vi "保存文件头.vi"(0 "error in (no error)":errorcluster caption="错误输入（无错误）", 1 "转角起点":dbl, 2 "转角终点":dbl, 3 "转角速度":dbl, 5 "实际备注数组":string[](array[string]), 7 "数据存储路径":path, 9 "采样率":u32, 11 "测试类型":dbl, 12 "单位":string, 13 "气压":dbl) -> (4 "error out":errorcluster caption="错误输出", 6 "引用句柄输出":refnum<file>, 15 "实际存储路径":path caption="新建文件路径（取消时为非法路径）")   [LabVIEW 2016]
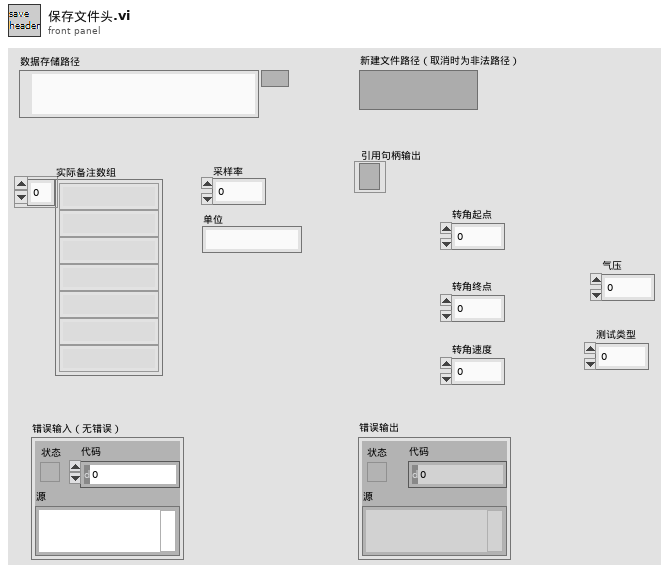
[diagram p1: front panel]
types:
  T1 = enum16{"open", "replace", "create", "open or create", "replace or create", "replace or create with confirmation"}
  T2 = cluster{"seconds since 1Jan1904":timestamp, "采样率":u32, "单位":string, "实际备注数组":string[], "转角终点":dbl, "转角起点":dbl, "转角速度":dbl, "测试类型":dbl, "气压":dbl}
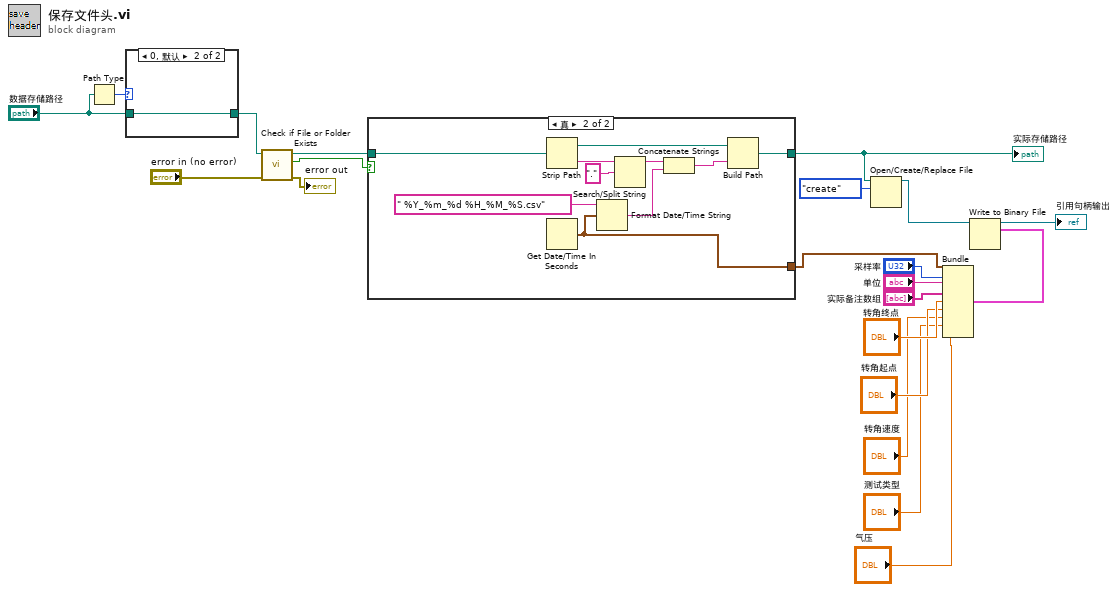
[diagram p0: block diagram]
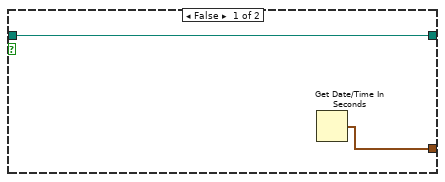
[diagram p2: hidden frame]
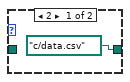
[diagram p3: hidden frame]
diagram:
  n1 = Path Type(1:"数据存储路径") -> (0:w21:i16)
  n2 = case shown="0, 默认" w21 {
    tunnel: "数据存储路径" -> [_ w23]
    tunnel: [path "c:/data.csv" w23] -> w17
    frame 2 {
    }
    frame 0, Default {
    }
  }
  n3 = call <vilib>:"Check if File or Folder Exists.vi"("error in (no error)"="error in (no error)", "path"=w17) -> ("error out"=→"error out":errorcluster, "file or folder exists?"=w18:bool, "dup path"=w19:path)  [unwired: 7 in]
  n4 = case shown="真" w18 {
    tunnel: w19 -> [w25 w35]
    tunnel: [w25 w27] -> w14
    tunnel: [w24 w26] -> w8
    frame False {
      n5 = Get Date/Time In Seconds() -> (seconds since 1Jan1904=w24:timestamp)
    }
    frame True {
      n6 = Strip Path(path=w35) -> (stripped path=w29:path, name=w32:string)
      n7 = Get Date/Time In Seconds() -> (seconds since 1Jan1904=w26:timestamp)
      n8 = Format Date/Time String(time format string (%c)=" %Y_%m_%d %H_%M_%S.csv" ("时间格式字符串(%c)"), seconds (now)=w26) -> (date/time string=w33:string)  [unwired: 1 in]
      n9 = Search/Split String(string=w32, search string/char (-)="." ("搜索字符串/字符(-)")) -> (substring before match=w30:string)  [unwired: 1 in, 2 out]
      n10 = Concatenate Strings(w30, w33) -> (w28:string)
      n11 = Build Path(base path=w29, name or relative path=w28) -> (appended path=w27:path)
    }
  }
  "实际存储路径" <- w14
  n12 = Open/Create/Replace File(file path (use dialog)=w14, operation (0:open)=T1."create" ("操作(0:open)")) -> (refnum out=w7:refnum<file>)  [unwired: 4 in, 2 out]
  n13 = Bundle("seconds since 1Jan1904"=w8, "采样率"="采样率", "单位"="单位", "实际备注数组"="实际备注数组", "转角终点"="转角终点", "转角起点"="转角起点", "转角速度"="转角速度", "测试类型"="测试类型", "气压"="气压") -> (w9:T2)  [unwired: 1 in]
  n14 = Write to Binary File(file (use dialog)=w7, data=w9) -> (refnum out=→"引用句柄输出":refnum<file>)  [unwired: 4 in, 2 out]
